vi "Parse First Tag Header.vi"(8 "error in (no error)":errorcluster, 10 "Flattened Linked List":string, 11 "XML in":refnum<class "XML.lvclass">) -> (0 "error out":errorcluster, 2 "Flattened Linked List After Tag":string, 3 "XML out":refnum<class "XML.lvclass">)   [LabVIEW 2020, in "XML.lvlib" / "XML.lvclass"]
uses:
  <vilib>/gpm_packages/@cs/persistence/source/XML/XML.lvclass
  <vilib>/gpm_packages/@cs/persistence/source/XML/XML.lvclass/XML.ctl
  <vilib>/Utility/error.llb/Error Cluster From Error Code.vi
  <vilib>/ErrorRing/Error Ring.xnode
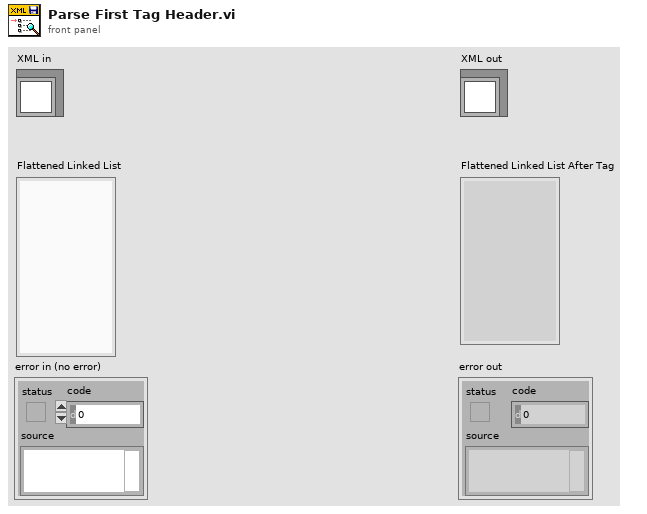
[diagram p1: front panel]
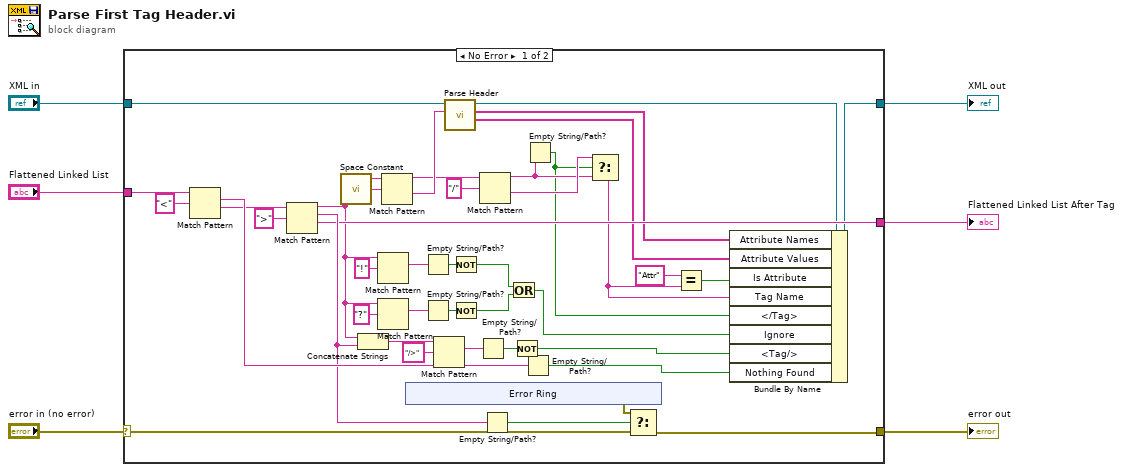
[diagram p0: block diagram]
diagram:
  n1 = case shown="No Error" "error in (no error)" {
    selector: "error in (no error)" -> [w23 w54]
    tunnel: "Flattened Linked List" -> [w31 _]
    tunnel: [w30 _] -> w5
    tunnel: "XML in" -> [w21 w55]
    tunnel: [w28 w55] -> w3
    tunnel: [w22 w54] -> w1
    frame No Error {
      n2 = Match Pattern(string=w31, regular expression="<") -> (match substring=w46:string, after substring=w34:string)  [unwired: 1 in, 2 out]
      n3 = Match Pattern(string=w34, regular expression=">") -> (before substring=w18:string, match substring=w42:string, after substring=w30:string)  [unwired: 1 in, 1 out]
      n4 = call <vilib>:"Space Constant.vi"() -> ("String"=w19:string)
      n5 = Concatenate Strings(w18, w42) -> (w41:string)
      n6 = Match Pattern(string=w18, regular expression="!") -> (match substring=w36:string)  [unwired: 1 in, 3 out]
      n7 = Match Pattern(string=w18, regular expression="?") -> (match substring=w39:string)  [unwired: 1 in, 3 out]
      n8 = Match Pattern(string=w18, regular expression=w19) -> (before substring=w13:string, after substring=w17:string)  [unwired: 1 in, 2 out]
      n9 = xnode "Error Ring"() -> ("error out"=w24:errorcluster)
      n10 = Empty String/Path?(string/path=w36) -> (empty?=w37:bool)
      n11 = Empty String/Path?(string/path=w39) -> (empty?=w38:bool)
      n12 = Match Pattern(string=w41, regular expression="/>") -> (match substring=w44:string)  [unwired: 1 in, 3 out]
      n13 = call-dynamic "Parse Header.vi"("Header"=w17, "XML in"=w21) -> ("Value"=w11:string[], "Name"=w10:string[], "XML out"=w20:refnum<class "XML.lvclass">)  [unwired: 7 in]
      n14 = Not(x=w37) -> (.not. x?=w32:bool)
      n15 = Not(x=w38) -> (.not. x?=w33:bool)
      n16 = Empty String/Path?(string/path=w44) -> (empty?=w43:bool)
      n17 = Match Pattern(string=w13, regular expression="/") -> (before substring=w14:string, after substring=w15:string)  [unwired: 1 in, 2 out]
      n18 = Empty String/Path?(string/path=w42) -> (empty?=w25:bool)
      n19 = Or(x=w32, y=w33) -> (x .or. y?=w26:bool)
      n20 = Not(x=w43) -> (.not. x?=w27:bool)
      n21 = Empty String/Path?(string/path=w46) -> (empty?=w29:bool)
      n22 = Empty String/Path?(string/path=w14) -> (empty?=w12:bool)
      n23 = Select(t=w15, s=w12, f=w14) -> (s? t:f=w9:string)
      n24 = Select(t=w24, s=w25, f=w23) -> (s? t:f=w22:errorcluster)
      n25 = Equal?(x="Attr", y=w9) -> (x = y?=w7:bool)
      n26 = Bundle By Name(cluster=w20, "Attribute Names"=w10, "Attribute Values"=w11, "Is Attribute"=w7, "Tag Name"=w9, "</Tag>"=w12, "Ignore"=w26, "<Tag/>"=w27, "Nothing Found"=w29) -> (w28:refnum<class "XML.lvclass">)
    }
    frame Error {
    }
  }
  "error out" <- w1
  "XML out" <- w3
  "Flattened Linked List After Tag" <- w5
